vi "UUT Test Info Insert Data.vi"(11 "Sequence Context":T1) -> (0 "error out":errorcluster)   [LabVIEW 2023, in "HardwareAbstractionLayer_LVOOP.lvlib" / "Report.lvclass"]
uses:
  Report.lvclass
  <vilib>/addons/TestStand/_TSLegacy.llb/LabVIEW Test - Sequence Context.ctl
  Control/UUT Test Info.ctl
  Control/All Log Details.ctl
  Control/FE FRAME LOG.ctl
  Control/FF FRAME LOG.ctl
  Control/LIMIT TABLE.ctl
  Control/ERROR LOG APPEND.ctl
  Control/ERROR LOG.ctl
  Control/FA FRAME LOG.ctl
  Control/TEST RESULT LOG APPEND.ctl
  Control/TEST RESULT LOG.ctl
  Control/SYSTEM LOG.ctl
  Control/Temperature LOG.ctl
  Control/POWER STATUS.ctl
  Control/CYCLE_DURATION_LOG.ctl
  <vilib>/addons/TestStand/_TSUtility.llb/TestStand - Get Property Value (String).vi
  <vilib>/addons/TestStand/_TSUtility.llb/TestStand - Get Property Value (Numeric Array {Signed 16-bit Integer}).vi
  <vilib>/addons/TestStand/_TSUtility.llb/TestStand - Get Property Value (Number {Signed 32-bit Integer}).vi
  Report.lvclass/Report.ctl
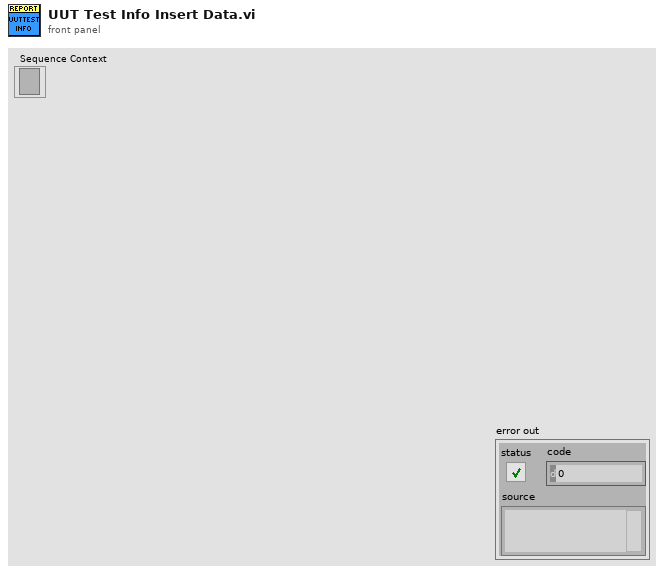
[diagram p1: front panel]
types:
  T1 = typedef "LabVIEW Test - Sequence Context.ctl" = refnum<k7>
  T2 = typedef "HardwareAbstractionLayer_LVOOP.lvlib/Report.lvclass/All Log Details.ctl" = cluster{"UUT_TEST_INFO":T3, "FE_FRAME_LOG":T4, "FF_FRAME_LOG":T5, "LIMIT_TABLE":T6, "ERROR LOG Append":T7, "FA_FRAME_LOG":T9, "Socket No":u16, "TEST RESULT LOG Append":T10, "SYSTEM_LOG":T12, "Temperature log":T13, "POWER_STATUS":T14, "CYCLE_DURATION_LOG":T15}
  T3 = typedef "HardwareAbstractionLayer_LVOOP.lvlib/Report.lvclass/UUT Test Info.ctl" = cluster{"ID":string, "STATION_ID":string, "TEST_SOCKET_INDEX":string, "UUT_SERIAL_NUMBER":string, "TSW_VER":string, "VAL_SW_VER":string, "PROJECT_NAME":string, "PRODUCT_NAME":string, "PRODUCT_VARIANT":string, "TEST_NAME":string, "TEST_PHASE":string, "TEST_DESCRIPTION":string, "TEMP_CHAMBER_NAME":string, "START_DATE_TIME":string, "STOP_DATE_TIME ":string, "START_CYCLE_COUNT":string, "STOP_CYCLE_COUNT":string, "EXECUTION_TIME":string, "UUT_STATUS":string, "UUT_ERROR_CODE":string, "UUT_ERROR_MESSAGE":string, "TEST_SEQUENCE":string}
  T4 = typedef "HardwareAbstractionLayer_LVOOP.lvlib/Report.lvclass/FE FRAME LOG.ctl" = cluster{"ID":string, "UUT_TEST_INFO":string, "DATE_TIME":string, "CYCLE_NUMBER":string, "TEST_MODE":string, "CHAMBER_TEMP":string, "CAN_FRAME_RX":string, "Test Mode":u32, "LV_PPS_VOLTAGE":string, "LV_PPS_CURRENT":string, "HV_PPS_VOLTAGE":string, "HV_PPS_CURRENT":string, "SOCKET_NUMBER":string, "CAN_FRAME_RX_NO_OFF_BYTE":string}
  T5 = typedef "HardwareAbstractionLayer_LVOOP.lvlib/Report.lvclass/FF FRAME LOG.ctl" = cluster{"ID":string, "UUT_TEST_INFO":string, "DATE_TIME":string, "CYCLE_NUMBER":string, "TEST_MODE":string, "CAN_FRAME_RX":string, "CHAMBER_TEMP":string, "TestMode":u32, "SOCKET_NUMBER":string, "CAN_FRAME_RX_NO_OFF_BYTE":string}
  T6 = typedef "HardwareAbstractionLayer_LVOOP.lvlib/Report.lvclass/LIMIT TABLE.ctl" = cluster{"ID":string, "PRODUCT_NAME":string, "PRODUCT_VARIANT":string, "TEST_MODE":string, "PARAMETER_NAME":string, "COMPARISON_TYPE":string, "LOW_LIMIT":string, "HIGH_LIMIT":string, "UNIT":string, "ERROR_MESSSAGE":string, "SEVERITY":string}
  T7 = typedef "HardwareAbstractionLayer_LVOOP.lvlib/Report.lvclass/ERROR LOG APPEND.ctl" = T8[]
  T8 = typedef "HardwareAbstractionLayer_LVOOP.lvlib/Report.lvclass/ERROR LOG.ctl" = cluster{"ID":string, "UUT_TEST_INFO":string, "DATE_TIME":string, "CYCLE_NUMBER":string, "TEST_MODE":string, "SIGNAL_NAME":string, "SIGNAL_VALUE":string, "UNIT":string, "COMPARISON_VALUE":string, "ERROR_MESSAGE":string, "FRAME_TYPE":string, "LIMITID":string, "SOCKET_NUMBER":string}
  T9 = typedef "HardwareAbstractionLayer_LVOOP.lvlib/Report.lvclass/FA FRAME LOG.ctl" = cluster{"UUT_TEST_INFO":string, "CAN_FRAME_RX":string, "CAN_FRAME_RX_NO_OFF_BYTE":string}
  T10 = typedef "HardwareAbstractionLayer_LVOOP.lvlib/Report.lvclass/TEST RESULT LOG APPEND.ctl" = T11[]
  T11 = typedef "HardwareAbstractionLayer_LVOOP.lvlib/Report.lvclass/TEST RESULT LOG.ctl" = cluster{"ID":string, "UUT_TEST_INFO":string, "DATE_TIME":string, "CYCLE_NUMBER":string, "TEST_MODE":string, "SIGNAL_NAME":string, "SIGNAL_VALUE":string, "COMPARISON_VALUE":string, "ERROR_MESSAGE":string, "FRAME_TYPE":string, "LIMITID":string, "TEST_RESULT":string, "SOCKET_NUMBER":string}
  T12 = typedef "HardwareAbstractionLayer_LVOOP.lvlib/Report.lvclass/SYSTEM LOG.ctl" = cluster{"ID ":string, "DATE_TIME":string, "CYCLE_NUMBER":string, "TEST_MODE":string, "ERROR_MESSAGE":string}
  T13 = typedef "HardwareAbstractionLayer_LVOOP.lvlib/Report.lvclass/Temperature LOG.ctl" = cluster{"TEST_MODE":string, "CYCLE_NUMBER":string, "TEMPERATURE":cluster{"LV_PPS_TEMPERATURE":dbl, "HV_PPS1_TEMPERATURE":dbl, "HV_PPS2_TEMPERATURE":dbl, "HV_PPS3_TEMPERATURE":dbl, "HV_PPS4_TEMPERATURE":dbl, "HV_PPS5_TEMPERATURE":dbl, "HV_PPS6_TEMPERATURE":dbl, "CHAMBER_TEMPERATURE":dbl, "LOAD_U1_TEMPERATURE":dbl, "LOAD_V1_TEMPERATURE":dbl, "LOAD_W1_TEMPERATURE":dbl, "LOAD_U2_TEMPERATURE":dbl, "LOAD_V2_TEMPERATURE":dbl, "LOAD_W2_TEMPERATURE":dbl, "LOAD_U3_TEMPERATURE":dbl, "LOAD_V3_TEMPERATURE":dbl, "LOAD_W3_TEMPERATURE":dbl}, "Temperature Inrange":cluster{"LVPPS_Trip?":bool, "HVPPS1_Trip?":bool, "HVPPS2_Trip?":bool, "HVPPS3_Trip?":bool, "HVPPS4_Trip?":bool, "HVPPS5_Trip?":bool, "HVPPS6_Trip?":bool, "Chamber_Trip?":bool}}
  T14 = typedef "HardwareAbstractionLayer_LVOOP.lvlib/Report.lvclass/POWER STATUS.ctl" = cluster{"TEST_MODE":string, "CYCLE_NUMBER":string, "TYPE_POWER":string, "STATE":string}
  T15 = typedef "HardwareAbstractionLayer_LVOOP.lvlib/Report.lvclass/CYCLE_DURATION_LOG.ctl" = cluster{"CYCLE_NUMBER":string}
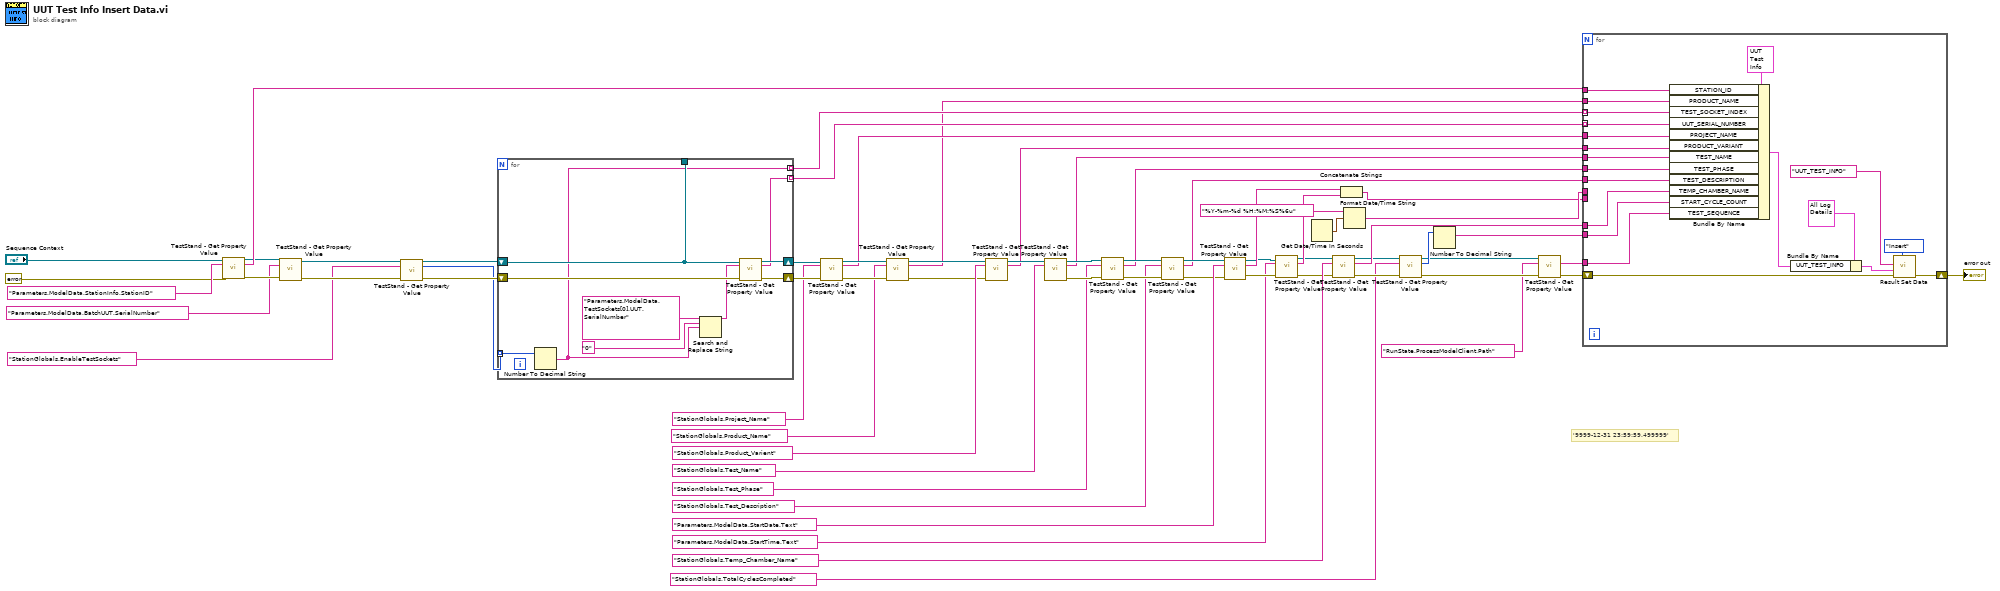
[diagram p0: block diagram]
diagram:
  # "'9999-12-31 23:59:59.499999'"
  n1 = call-poly <vilib>:"TestStand - Get Property Value.vi"("Sequence Context In"="Sequence Context", "Lookup String"="Parameters.ModelData.StationInfo.StationID", "error in (no error)"=errorcluster {"status"=FALSE, "code"=0, "source"=""} ("error in")) -> ("Sequence Context Out"=w41:refnum<k7>, "Value"=w61:string, "error out"=w62:errorcluster)  [unwired: 10 in]
  n2 = call-poly <vilib>:"TestStand - Get Property Value.vi"("Sequence Context In"=w41, "Lookup String"="Parameters.ModelData.BatchUUT.SerialNumber", "error in (no error)"=w62) -> ("Sequence Context Out"=w42:refnum<k7>, "error out"=w59:errorcluster)  [unwired: 10 in, 1 out]
  n3 = call-poly <vilib>:"TestStand - Get Property Value.vi"("Sequence Context In"=w42, "Lookup String"="StationGlobals.EnableTestSockets") -> ("Sequence Context Out"=w43:refnum<k7>, "Value"=w39:i16[])  [unwired: 11 in, 1 out]
  n4 = for {
    tunnel: [w65] -> w58 mode=indexing
    shift-right: [w71] -> w56
    shift-left: w59 -> [w74]
    shift-right: [w72] -> w44
    shift-left: w43 -> [w73]
    tunnel: [w67] -> w57 mode=indexing
    tunnel: [w73] -> _
    tunnel: w39 -> [w66] mode=indexing
    n5 = Number To Decimal String(number=w66) -> (decimal integer string=w65:string)  [unwired: 1 in]
    n6 = Search and Replace String(input string="Parameters.ModelData.TestSockets[0].UUT.SerialNumber" ("Lookup String"), search string="0", replace string=w65) -> (result string=w68:string)  [unwired: 5 in, 3 out]
    n7 = call-poly <vilib>:"TestStand - Get Property Value.vi"("Sequence Context In"=w73, "Lookup String"=w68, "error in (no error)"=w74) -> ("Sequence Context Out"=w72:refnum<k7>, "Value"=w67:string, "error out"=w71:errorcluster)  [unwired: 10 in]
  }
  n8 = call-poly <vilib>:"TestStand - Get Property Value.vi"("Sequence Context In"=w44, "Lookup String"="StationGlobals.Project_Name", "error in (no error)"=w56) -> ("Sequence Context Out"=w21:refnum<k7>, "Value"=w16:string, "error out"=w19:errorcluster)  [unwired: 10 in]
  n9 = call-poly <vilib>:"TestStand - Get Property Value.vi"("Sequence Context In"=w21, "Lookup String"="StationGlobals.Product_Name", "error in (no error)"=w19) -> ("Sequence Context Out"=w20:refnum<k7>, "Value"=w11:string, "error out"=w18:errorcluster)  [unwired: 10 in]
  n10 = call-poly <vilib>:"TestStand - Get Property Value.vi"("Sequence Context In"=w20, "Lookup String"="StationGlobals.Product_Varient", "error in (no error)"=w18) -> ("Sequence Context Out"=w36:refnum<k7>, "Value"=w26:string)  [unwired: 10 in, 1 out]
  n11 = call-poly <vilib>:"TestStand - Get Property Value.vi"("Sequence Context In"=w36, "Lookup String"="StationGlobals.Test_Name") -> ("Sequence Context Out"=w35:refnum<k7>, "Value"=w25:string, "error out"=w34:errorcluster)  [unwired: 11 in]
  n12 = call-poly <vilib>:"TestStand - Get Property Value.vi"("Sequence Context In"=w35, "Lookup String"="StationGlobals.Test_Phase", "error in (no error)"=w34) -> ("Sequence Context Out"=w31:refnum<k7>, "Value"=w24:string, "error out"=w29:errorcluster)  [unwired: 10 in]
  n13 = call-poly <vilib>:"TestStand - Get Property Value.vi"("Sequence Context In"=w31, "Lookup String"="StationGlobals.Test_Description", "error in (no error)"=w29) -> ("Sequence Context Out"=w30:refnum<k7>, "Value"=w23:string, "error out"=w28:errorcluster)  [unwired: 10 in]
  n14 = call-poly <vilib>:"TestStand - Get Property Value.vi"("Sequence Context In"=w30, "Lookup String"="Parameters.ModelData.StartDate.Text", "error in (no error)"=w28) -> ("Sequence Context Out"=w45:refnum<k7>, "Value"=w49:string, "error out"=w52:errorcluster)  [unwired: 10 in]
  n15 = call-poly <vilib>:"TestStand - Get Property Value.vi"("Sequence Context In"=w45, "Lookup String"="Parameters.ModelData.StartTime.Text", "error in (no error)"=w52) -> ("Sequence Context Out"=w46:refnum<k7>, "Value"=w48:string, "error out"=w50:errorcluster)  [unwired: 10 in]
  n16 = Get Date/Time In Seconds() -> (seconds since 1Jan1904=w14:timestamp)
  n17 = call-poly <vilib>:"TestStand - Get Property Value.vi"("Sequence Context In"=w46, "Lookup String"="StationGlobals.Temp_Chamber_Name", "error in (no error)"=w50) -> ("Sequence Context Out"=w9:refnum<k7>, "Value"=w22:string, "error out"=w10:errorcluster)  [unwired: 10 in]
  n18 = Concatenate Strings(w49, w48) -> (w12:string)
  n19 = Format Date/Time String(time format string (%c)="%Y-%m-%d %H:%M:%S%6u", seconds (now)=w14) -> (date/time string=w13:string)  [unwired: 1 in]
  n20 = call-poly <vilib>:"TestStand - Get Property Value.vi"("Sequence Context In"=w9, "Lookup String"="StationGlobals.TotalCyclesCompleted", "error in (no error)"=w10) -> ("Sequence Context Out"=w3:refnum<k7>, "Value"=w8:i32, "error out"=w5:errorcluster)  [unwired: 10 in]
  n21 = Number To Decimal String(number=w8) -> (decimal integer string=w6:string)  [unwired: 1 in]
  n22 = call-poly <vilib>:"TestStand - Get Property Value.vi"("Sequence Context In"=w3, "Lookup String"="RunState.ProcessModelClient.Path", "error in (no error)"=w5) -> ("Value"=w1:string, "error out"=w4:errorcluster)  [unwired: 10 in, 1 out]
  n23 = for {
    tunnel: w61 -> [w89]
    tunnel: w11 -> [w88]
    tunnel: w58 -> [w87] mode=indexing
    tunnel: w57 -> [w86] mode=indexing
    tunnel: w16 -> [w85]
    tunnel: w13 -> [_]
    tunnel: w22 -> [w84]
    shift-right: [w82] -> w38
    shift-left: w4 -> [w83]
    tunnel: w26 -> [w81]
    tunnel: w25 -> [w80]
    tunnel: w24 -> [w79]
    tunnel: w23 -> [w78]
    tunnel: w12 -> [_]
    tunnel: w6 -> [w77]
    tunnel: w1 -> [w75]
    n24 = Bundle By Name(cluster=T3 {"ID"="", "STATION_ID"="", "TEST_SOCKET_INDEX"="", "UUT_SERIAL_NUMBER"="", "TSW_VER"="", "VAL_SW_VER"="", "PROJECT_NAME"="", "PRODUCT_NAME"="", "PRODUCT_VARIANT"="", "TEST_NAME"="", "TEST_PHASE"="", "TEST_DESCRIPTION"="", "TEMP_CHAMBER_NAME"="", "START_DATE_TIME"="", "STOP_DATE_TIME "="", "START_CYCLE_COUNT"="", "STOP_CYCLE_COUNT"="", "EXECUTION_TIME"="", "UUT_STATUS"="", "UUT_ERROR_CODE"="", "UUT_ERROR_MESSAGE"="", "TEST_SEQUENCE"=""} ("UUT_TEST_INFO"), "STATION_ID"=w89, "PRODUCT_NAME"=w88, "TEST_SOCKET_INDEX"=w87, "UUT_SERIAL_NUMBER"=w86, "PROJECT_NAME"=w85, "PRODUCT_VARIANT"=w81, "TEST_NAME"=w80, "TEST_PHASE"=w79, "TEST_DESCRIPTION"=w78, "TEMP_CHAMBER_NAME"=w84, "START_CYCLE_COUNT"=w77, "TEST_SEQUENCE"=w75) -> (w91:T3)
    n25 = Bundle By Name(cluster=T2 {"UUT_TEST_INFO"={"ID"="", "STATION_ID"="", "TEST_SOCKET_INDEX"="", "UUT_SERIAL_NUMBER"="", "TSW_VER"="", "VAL_SW_VER"="", "PROJECT_NAME"="", "PRODUCT_NAME"="", "PRODUCT_VARIANT"="", "TEST_NAME"="", "TEST_PHASE"="", "TEST_DESCRIPTION"="", "TEMP_CHAMBER_NAME"="", "START_DATE_TIME"="", "STOP_DATE_TIME "="", "START_CYCLE_COUNT"="", "STOP_CYCLE_COUNT"="", "EXECUTION_TIME"="", "UUT_STATUS"="", "UUT_ERROR_CODE"="", "UUT_ERROR_MESSAGE"="", "TEST_SEQUENCE"=""}, "FE_FRAME_LOG"={"ID"="", "UUT_TEST_INFO"="", "DATE_TIME"="", "CYCLE_NUMBER"="", "TEST_MODE"="", "CHAMBER_TEMP"="", "CAN_FRAME_RX"="", "Test Mode"=0, "LV_PPS_VOLTAGE"="", "LV_PPS_CURRENT"="", "HV_PPS_VOLTAGE"="", "HV_PPS_CURRENT"="", "SOCKET_NUMBER"="", "CAN_FRAME_RX_NO_OFF_BYTE"=""}, "FF_FRAME_LOG"={"ID"="", "UUT_TEST_INFO"="", "DATE_TIME"="", "CYCLE_NUMBER"="", "TEST_MODE"="", "CAN_FRAME_RX"="", "CHAMBER_TEMP"="", "TestMode"=0, "SOCKET_NUMBER"="", "CAN_FRAME_RX_NO_OFF_BYTE"=""}, "LIMIT_TABLE"={"ID"="", "PRODUCT_NAME"="", "PRODUCT_VARIANT"="", "TEST_MODE"="", "PARAMETER_NAME"="", "COMPARISON_TYPE"="", "LOW_LIMIT"="", "HIGH_LIMIT"="", "UNIT"="", "ERROR_MESSSAGE"="", "SEVERITY"=""}, "ERROR LOG Append"=[], "FA_FRAME_LOG"={"UUT_TEST_INFO"="", "CAN_FRAME_RX"="", "CAN_FRAME_RX_NO_OFF_BYTE"=""}, "Socket No"=1, "TEST RESULT LOG Append"=[], "SYSTEM_LOG"={"ID "="", "DATE_TIME"="", "CYCLE_NUMBER"="", "TEST_MODE"="", "ERROR_MESSAGE"=""}, "Temperature log"={"TEST_MODE"="", "CYCLE_NUMBER"="", "TEMPERATURE"={"LV_PPS_TEMPERATURE"=0.0, "HV_PPS1_TEMPERATURE"=0.0, "HV_PPS2_TEMPERATURE"=0.0, "HV_PPS3_TEMPERATURE"=0.0, "HV_PPS4_TEMPERATURE"=0.0, "HV_PPS5_TEMPERATURE"=0.0, "HV_PPS6_TEMPERATURE"=0.0, "CHAMBER_TEMPERATURE"=0.0, "LOAD_U1_TEMPERATURE"=0.0, "LOAD_V1_TEMPERATURE"=0.0, "LOAD_W1_TEMPERATURE"=0.0, "LOAD_U2_TEMPERATURE"=0.0, "LOAD_V2_TEMPERATURE"=0.0, "LOAD_W2_TEMPERATURE"=0.0, "LOAD_U3_TEMPERATURE"=0.0, "LOAD_V3_TEMPERATURE"=0.0, "LOAD_W3_TEMPERATURE"=0.0}, "Temperature Inrange"={"LVPPS_Trip?"=FALSE, "HVPPS1_Trip?"=FALSE, "HVPPS2_Trip?"=FALSE, "HVPPS3_Trip?"=FALSE, "HVPPS4_Trip?"=FALSE, "HVPPS5_Trip?"=FALSE, "HVPPS6_Trip?"=FALSE, "Chamber_Trip?"=FALSE}}, "POWER_STATUS"={"TEST_MODE"="", "CYCLE_NUMBER"="", "TYPE_POWER"="", "STATE"=""}, "CYCLE_DURATION_LOG"={"CYCLE_NUMBER"=""}} ("Set Data"), "UUT_TEST_INFO"=w91) -> (w90:T2)
    n26 = call "Result Set Data.vi"("error in"=w83, "Set Data"=w90, "Table Name"="UUT_TEST_INFO", "Action"=enum16{"Insert", "Update"}."Insert") -> ("error out"=w82:errorcluster)  [unwired: 7 in]
  }
  "error out" <- w38
